vi "ZoneRed to ZoneBlue.vi"   [LabVIEW 2019]
uses:
  Global Var.vi
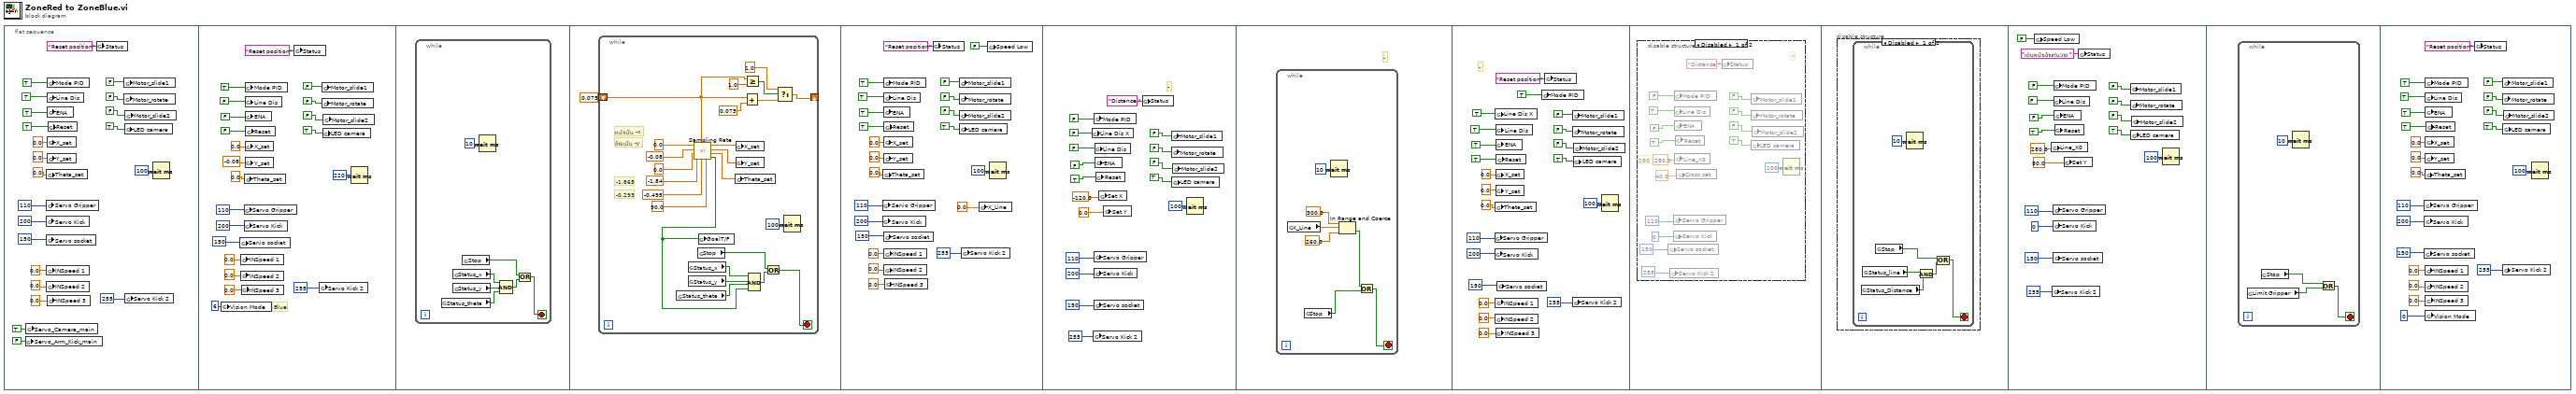
[diagram p0: block diagram]
diagram:
  n1 = flat-sequence {
    frame #0 {
      n2 = global write "Global Var.vi" "Servo_Arm_Kick_main"(FALSE ("Mode PID")) -> ()
      n3 = global write "Global Var.vi" "Servo_Camera_main"(TRUE ("Mode PID")) -> ()
      n4 = global write "Global Var.vi" "Servo Gripper"(u8 110 ("Servo Camera")) -> ()
      n5 = global write "Global Var.vi" "Servo Kick"(u8 200 ("Servo Camera")) -> ()
      n6 = global write "Global Var.vi" "Servo socket"(u8 150 ("Servo Camera")) -> ()
      n7 = global write "Global Var.vi" "Theta_set"(0.0 ("Theta_set")) -> ()
      n8 = global write "Global Var.vi" "INSpeed 1"(0.0 ("X_set")) -> ()
      n9 = global write "Global Var.vi" "INSpeed 2"(0.0 ("Y_set")) -> ()
      n10 = global write "Global Var.vi" "Mode PID"(TRUE ("Mode PID")) -> ()
      n11 = global write "Global Var.vi" "Line Dis"(TRUE ("Mode PID")) -> ()
      n12 = global write "Global Var.vi" "ENA"(TRUE ("ENA")) -> ()
      n13 = global write "Global Var.vi" "X_set"(0.0 ("X_set")) -> ()
      n14 = global write "Global Var.vi" "Y_set"(0.0 ("Y_set")) -> ()
      n15 = global write "Global Var.vi" "INSpeed 3"(0.0 ("Theta_set")) -> ()
      n16 = global write "Global Var.vi" "Reset"(TRUE ("ENA")) -> ()
      n17 = global write "Global Var.vi" "Status"("Reset position" ("Status")) -> ()
      n18 = global write "Global Var.vi" "Motor_slide1"(FALSE ("Mode PID")) -> ()
      n19 = global write "Global Var.vi" "Motor_rotate"(FALSE ("ENA")) -> ()
      n20 = global write "Global Var.vi" "LED camera"(TRUE ("LED camera")) -> ()
      n21 = global write "Global Var.vi" "Motor_slide2"(FALSE ("ENA")) -> ()
      n22 = global write "Global Var.vi" "Servo Kick 2"(u8 255 ("Servo Camera")) -> ()
      n23 = Wait (ms)(milliseconds to wait=u32 100) -> ()  [unwired: 1 out]
    }
    frame #1 {
      # "Blue"
      n24 = global write "Global Var.vi" "Vision Mode"(i16 6 ("Vision Mode")) -> ()
      n25 = global write "Global Var.vi" "Servo socket"(u8 150 ("Servo Camera")) -> ()
      n26 = global write "Global Var.vi" "INSpeed 1"(0.0 ("X_set")) -> ()
      n27 = global write "Global Var.vi" "INSpeed 2"(0.0 ("Y_set")) -> ()
      n28 = global write "Global Var.vi" "INSpeed 3"(0.0 ("Theta_set")) -> ()
      n29 = global write "Global Var.vi" "Servo Gripper"(u8 110 ("Servo Camera")) -> ()
      n30 = global write "Global Var.vi" "Servo Kick"(u8 200 ("Servo Camera")) -> ()
      n31 = global write "Global Var.vi" "Theta_set"(0.0 ("Theta_set")) -> ()
      n32 = global write "Global Var.vi" "Mode PID"(TRUE ("Mode PID")) -> ()
      n33 = global write "Global Var.vi" "Line Dis"(FALSE ("Mode PID")) -> ()
      n34 = global write "Global Var.vi" "ENA"(FALSE ("ENA")) -> ()
      n35 = global write "Global Var.vi" "X_set"(0.0 ("X_set")) -> ()
      n36 = global write "Global Var.vi" "Y_set"(-0.08 ("Y_set")) -> ()
      n37 = global write "Global Var.vi" "Reset"(FALSE ("ENA")) -> ()
      n38 = global write "Global Var.vi" "Status"("Reset position" ("Status")) -> ()
      n39 = global write "Global Var.vi" "Servo Kick 2"(u8 255 ("Servo Camera")) -> ()
      n40 = global write "Global Var.vi" "Motor_slide1"(FALSE ("Mode PID")) -> ()
      n41 = global write "Global Var.vi" "Motor_rotate"(FALSE ("ENA")) -> ()
      n42 = global write "Global Var.vi" "LED camera"(TRUE ("LED camera")) -> ()
      n43 = global write "Global Var.vi" "Motor_slide2"(FALSE ("ENA")) -> ()
      n44 = Wait (ms)(milliseconds to wait=u32 220) -> ()  [unwired: 1 out]
    }
    frame #2 {
      n45 = while {
        stop <- w46 stop-if-true
        n46 = global read "Global Var.vi" "Status_theta"() -> (w48:bool)
        n47 = global read "Global Var.vi" "Status_x"() -> (w49:bool)
        n48 = global read "Global Var.vi" "Status_y"() -> (w50:bool)
        n49 = global read "Global Var.vi" "Stop"() -> (w44:bool)
        n50 = Wait (ms)(milliseconds to wait=u32 10) -> ()  [unwired: 1 out]
        n51 = Compound Arithmetic op=AND(w49, w50, w48) -> (w45:bool)
        n52 = Or(x=w44, y=w45) -> (x .or. y?=w46:bool)
      }
    }
    frame #3 {
      n53 = while {
        shift-right: [w54] -> _
        shift-left: 0.075 -> [w52]
        stop <- w71 stop-if-true
        # "-0.293"
        # "-1.865"
        # "ซ้ายเป็น -y"
        # "หน้าเป็น -x"
        n54 = global read "Global Var.vi" "Status_theta"() -> (w73:bool)
        n55 = global read "Global Var.vi" "Status_x"() -> (w74:bool)
        n56 = global read "Global Var.vi" "Status_y"() -> (w75:bool)
        n57 = call "Sampling Rate.vi"("input a1"=90.0, "input y1"=-0.495, "T(0-1)"=w52, "input x1"=-1.84, "input a0"=0.0, "input y0"=-0.08, "input x0"=0.0) -> ("GoalT/F"=w59:bool, "a_output"=w66:dbl, "y_output"=w67:dbl, "x_output"=w68:dbl)  [unwired: 1 in]
        n58 = global read "Global Var.vi" "Stop"() -> (w69:bool)
        n59 = global write "Global Var.vi" "GoalT/F"(w59) -> ()
        n60 = global write "Global Var.vi" "Theta_set"(w66) -> ()
        n61 = global write "Global Var.vi" "X_set"(w68) -> ()
        n62 = global write "Global Var.vi" "Y_set"(w67) -> ()
        n63 = Add(x=w52, y=0.075) -> (x+y=w57:dbl)
        n64 = Greater Or Equal?(x=w52, y=1.0) -> (x >= y?=w56:bool)
        n65 = Compound Arithmetic op=AND(w74, w75, w73, w59) -> (w70:bool)
        n66 = Or(x=w69, y=w70) -> (x .or. y?=w71:bool)
        n67 = Select(t=1.0, s=w56, f=w57) -> (s? t:f=w54:dbl)
        n68 = Wait (ms)(milliseconds to wait=u32 100) -> ()  [unwired: 1 out]
      }
    }
    frame #4 {
      n69 = global write "Global Var.vi" "Servo Gripper"(u8 110 ("Servo Camera")) -> ()
      n70 = global write "Global Var.vi" "Servo Kick"(u8 200 ("Servo Camera")) -> ()
      n71 = global write "Global Var.vi" "Theta_set"(0.0 ("Theta_set")) -> ()
      n72 = global write "Global Var.vi" "Mode PID"(TRUE ("Mode PID")) -> ()
      n73 = global write "Global Var.vi" "Line Dis"(TRUE ("Mode PID")) -> ()
      n74 = global write "Global Var.vi" "ENA"(TRUE ("ENA")) -> ()
      n75 = global write "Global Var.vi" "X_set"(0.0 ("X_set")) -> ()
      n76 = global write "Global Var.vi" "Y_set"(0.0 ("Y_set")) -> ()
      n77 = global write "Global Var.vi" "Servo socket"(u8 150 ("Servo Camera")) -> ()
      n78 = global write "Global Var.vi" "Reset"(TRUE ("ENA")) -> ()
      n79 = global write "Global Var.vi" "INSpeed 1"(0.0 ("X_set")) -> ()
      n80 = global write "Global Var.vi" "INSpeed 2"(0.0 ("Y_set")) -> ()
      n81 = global write "Global Var.vi" "INSpeed 3"(0.0 ("Theta_set")) -> ()
      n82 = global write "Global Var.vi" "Status"("Reset position" ("Status")) -> ()
      n83 = global write "Global Var.vi" "Motor_slide1"(FALSE ("Mode PID")) -> ()
      n84 = global write "Global Var.vi" "Motor_rotate"(FALSE ("ENA")) -> ()
      n85 = global write "Global Var.vi" "Motor_slide2"(FALSE ("ENA")) -> ()
      n86 = global write "Global Var.vi" "LED camera"(TRUE ("LED camera")) -> ()
      n87 = global write "Global Var.vi" "Servo Kick 2"(u8 255 ("Servo Camera")) -> ()
      n88 = global write "Global Var.vi" "X_Line"(0.0 ("X_set")) -> ()
      n89 = global write "Global Var.vi" "Speed Low"(FALSE ("LED camera")) -> ()
      n90 = Wait (ms)(milliseconds to wait=u32 100) -> ()  [unwired: 1 out]
    }
    frame #5 {
      # "-"
      n91 = global write "Global Var.vi" "Line Dis X"(FALSE ("Mode PID")) -> ()
      n92 = global write "Global Var.vi" "Servo Kick 2"(u8 255 ("Servo Camera")) -> ()
      n93 = global write "Global Var.vi" "Mode PID"(FALSE ("Mode PID")) -> ()
      n94 = global write "Global Var.vi" "Servo Gripper"(u8 110 ("Servo Camera")) -> ()
      n95 = global write "Global Var.vi" "Servo Kick"(u8 200 ("Servo Camera")) -> ()
      n96 = global write "Global Var.vi" "Servo socket"(u8 150 ("Servo Camera")) -> ()
      n97 = global write "Global Var.vi" "Line Dis"(FALSE ("Mode PID")) -> ()
      n98 = global write "Global Var.vi" "ENA"(FALSE ("ENA")) -> ()
      n99 = global write "Global Var.vi" "Reset"(TRUE ("ENA")) -> ()
      n100 = global write "Global Var.vi" "Set X"(-120.0 ("Y_set")) -> ()
      n101 = global write "Global Var.vi" "Set Y"(0.0 ("Y_set")) -> ()
      n102 = global write "Global Var.vi" "Status"("Distance " ("Status")) -> ()
      n103 = global write "Global Var.vi" "Motor_slide1"(FALSE ("Mode PID")) -> ()
      n104 = global write "Global Var.vi" "Motor_rotate"(FALSE ("ENA")) -> ()
      n105 = global write "Global Var.vi" "LED camera"(TRUE ("LED camera")) -> ()
      n106 = global write "Global Var.vi" "Motor_slide2"(FALSE ("ENA")) -> ()
      n107 = Wait (ms)(milliseconds to wait=u32 100) -> ()  [unwired: 1 out]
    }
    frame #6 {
      # "-"
      n108 = while {
        stop <- w120 stop-if-true
        n109 = global read "Global Var.vi" "X_Line"() -> (w118:dbl)
        n110 = global read "Global Var.vi" "Stop"() -> (w119:bool)
        n111 = Wait (ms)(milliseconds to wait=u32 10) -> ()  [unwired: 1 out]
        n112 = In Range and Coerce(upper limit=300.0, x=w118, lower limit=260.0) -> (In Range?=w115:bool)  [unwired: 1 out]
        n113 = Or(x=w115, y=w119) -> (x .or. y?=w120:bool)
      }
    }
    frame #7 {
      # "-"
      n114 = global write "Global Var.vi" "Servo Gripper"(u8 110 ("Servo Camera")) -> ()
      n115 = global write "Global Var.vi" "Servo Kick"(u8 200 ("Servo Camera")) -> ()
      n116 = global write "Global Var.vi" "Line Dis X"(TRUE ("Mode PID")) -> ()
      n117 = global write "Global Var.vi" "Theta_set"(0.0 ("Theta_set")) -> ()
      n118 = global write "Global Var.vi" "INSpeed 1"(0.0 ("X_set")) -> ()
      n119 = global write "Global Var.vi" "INSpeed 2"(0.0 ("Y_set")) -> ()
      n120 = global write "Global Var.vi" "Line Dis"(TRUE ("Mode PID")) -> ()
      n121 = global write "Global Var.vi" "ENA"(TRUE ("ENA")) -> ()
      n122 = global write "Global Var.vi" "X_set"(0.0 ("X_set")) -> ()
      n123 = global write "Global Var.vi" "Y_set"(0.0 ("Y_set")) -> ()
      n124 = global write "Global Var.vi" "INSpeed 3"(0.0 ("Theta_set")) -> ()
      n125 = global write "Global Var.vi" "Reset"(TRUE ("ENA")) -> ()
      n126 = global write "Global Var.vi" "Servo socket"(u8 150 ("Servo Camera")) -> ()
      n127 = global write "Global Var.vi" "Mode PID"(TRUE ("Mode PID")) -> ()
      n128 = global write "Global Var.vi" "Status"("Reset position" ("Status")) -> ()
      n129 = global write "Global Var.vi" "Motor_slide1"(FALSE ("Mode PID")) -> ()
      n130 = global write "Global Var.vi" "Motor_rotate"(FALSE ("ENA")) -> ()
      n131 = global write "Global Var.vi" "Servo Kick 2"(u8 255 ("Servo Camera")) -> ()
      n132 = global write "Global Var.vi" "LED camera"(TRUE ("LED camera")) -> ()
      n133 = global write "Global Var.vi" "Motor_slide2"(FALSE ("ENA")) -> ()
      n134 = Wait (ms)(milliseconds to wait=u32 100) -> ()  [unwired: 1 out]
    }
    frame #8 {
      n135 = disable-structure shown="Disabled" {
        frame Disabled {
          # "280"
          # "*"
          n136 = global write "Global Var.vi" "Servo socket"(u8 150 ("Servo Camera")) -> ()
          n137 = global write "Global Var.vi" "Servo Kick 2"(u8 255 ("Servo Camera")) -> ()
          n138 = global write "Global Var.vi" "Servo Gripper"(u8 110 ("Servo Camera")) -> ()
          n139 = global write "Global Var.vi" "Servo Kick"(u8 0 ("Servo Camera")) -> ()
          n140 = global write "Global Var.vi" "Mode PID"(FALSE ("Mode PID")) -> ()
          n141 = global write "Global Var.vi" "Line Dis"(TRUE ("Mode PID")) -> ()
          n142 = global write "Global Var.vi" "ENA"(FALSE ("ENA")) -> ()
          n143 = global write "Global Var.vi" "Line_X0"(280.0 ("Y_set")) -> ()
          n144 = global write "Global Var.vi" "Reset"(TRUE ("ENA")) -> ()
          n145 = global write "Global Var.vi" "Cross set"(40.0 ("Y_set")) -> ()
          n146 = global write "Global Var.vi" "Status"("Distance " ("Status")) -> ()
          n147 = global write "Global Var.vi" "Motor_slide1"(FALSE ("Mode PID")) -> ()
          n148 = global write "Global Var.vi" "Motor_rotate"(FALSE ("ENA")) -> ()
          n149 = global write "Global Var.vi" "LED camera"(TRUE ("LED camera")) -> ()
          n150 = global write "Global Var.vi" "Motor_slide2"(FALSE ("ENA")) -> ()
          n151 = Wait (ms)(milliseconds to wait=u32 100) -> ()  [unwired: 1 out]
        }
        frame Enabled {
        }
      }
    }
    frame #9 {
      n152 = disable-structure shown="Disabled" {
        frame Disabled {
          n153 = while {
            stop <- w163 stop-if-true
            n154 = global read "Global Var.vi" "Status_Distance"() -> (w159:bool)
            n155 = global read "Global Var.vi" "Status_line"() -> (w160:bool)
            n156 = global read "Global Var.vi" "Stop"() -> (w162:bool)
            n157 = Wait (ms)(milliseconds to wait=u32 10) -> ()  [unwired: 1 out]
            n158 = And(x=w160, y=w159) -> (x .and. y?=w161:bool)
            n159 = Or(x=w162, y=w161) -> (x .or. y?=w163:bool)
          }
        }
        frame Enabled {
        }
      }
    }
    frame #10 {
      n160 = global write "Global Var.vi" "Speed Low"(FALSE ("LED camera")) -> ()
      n161 = global write "Global Var.vi" "Line_X0"(280.0 ("Y_set")) -> ()
      n162 = global write "Global Var.vi" "Servo Kick 2"(u8 255 ("Servo Camera")) -> ()
      n163 = global write "Global Var.vi" "Servo Gripper"(u8 110 ("Servo Camera")) -> ()
      n164 = global write "Global Var.vi" "Servo Kick"(u8 0 ("Servo Camera")) -> ()
      n165 = global write "Global Var.vi" "Servo socket"(u8 150 ("Servo Camera")) -> ()
      n166 = global write "Global Var.vi" "Mode PID"(FALSE ("Mode PID")) -> ()
      n167 = global write "Global Var.vi" "Line Dis"(FALSE ("Mode PID")) -> ()
      n168 = global write "Global Var.vi" "ENA"(FALSE ("ENA")) -> ()
      n169 = global write "Global Var.vi" "Reset"(TRUE ("ENA")) -> ()
      n170 = global write "Global Var.vi" "Set Y"(80.0 ("Y_set")) -> ()
      n171 = global write "Global Var.vi" "Status"("เดินหน้าเข้าแท่นวาง " ("Status")) -> ()
      n172 = global write "Global Var.vi" "Motor_slide1"(FALSE ("Mode PID")) -> ()
      n173 = global write "Global Var.vi" "Motor_rotate"(FALSE ("ENA")) -> ()
      n174 = global write "Global Var.vi" "LED camera"(TRUE ("LED camera")) -> ()
      n175 = global write "Global Var.vi" "Motor_slide2"(FALSE ("ENA")) -> ()
      n176 = Wait (ms)(milliseconds to wait=u32 100) -> ()  [unwired: 1 out]
    }
    frame #11 {
      n177 = while {
        stop <- w184 stop-if-true
        n178 = global read "Global Var.vi" "Limit Gripper"() -> (w182:bool)
        n179 = global read "Global Var.vi" "Stop"() -> (w183:bool)
        n180 = Wait (ms)(milliseconds to wait=u32 10) -> ()  [unwired: 1 out]
        n181 = Or(x=w183, y=w182) -> (x .or. y?=w184:bool)
      }
    }
    frame #12 {
      n182 = global write "Global Var.vi" "Servo Gripper"(u8 110 ("Servo Camera")) -> ()
      n183 = global write "Global Var.vi" "Servo Kick"(u8 200 ("Servo Camera")) -> ()
      n184 = global write "Global Var.vi" "Servo socket"(u8 150 ("Servo Camera")) -> ()
      n185 = global write "Global Var.vi" "Theta_set"(0.0 ("Theta_set")) -> ()
      n186 = global write "Global Var.vi" "INSpeed 1"(0.0 ("X_set")) -> ()
      n187 = global write "Global Var.vi" "INSpeed 2"(0.0 ("Y_set")) -> ()
      n188 = global write "Global Var.vi" "Mode PID"(TRUE ("Mode PID")) -> ()
      n189 = global write "Global Var.vi" "Line Dis"(TRUE ("Mode PID")) -> ()
      n190 = global write "Global Var.vi" "ENA"(TRUE ("ENA")) -> ()
      n191 = global write "Global Var.vi" "X_set"(0.0 ("X_set")) -> ()
      n192 = global write "Global Var.vi" "Y_set"(0.0 ("Y_set")) -> ()
      n193 = global write "Global Var.vi" "INSpeed 3"(0.0 ("Theta_set")) -> ()
      n194 = global write "Global Var.vi" "Vision Mode"(i16 0 ("Vision Mode")) -> ()
      n195 = global write "Global Var.vi" "Reset"(TRUE ("ENA")) -> ()
      n196 = global write "Global Var.vi" "Status"("Reset position" ("Status")) -> ()
      n197 = global write "Global Var.vi" "Motor_slide1"(FALSE ("Mode PID")) -> ()
      n198 = global write "Global Var.vi" "Motor_rotate"(FALSE ("ENA")) -> ()
      n199 = global write "Global Var.vi" "Servo Kick 2"(u8 255 ("Servo Camera")) -> ()
      n200 = global write "Global Var.vi" "LED camera"(TRUE ("LED camera")) -> ()
      n201 = global write "Global Var.vi" "Motor_slide2"(FALSE ("ENA")) -> ()
      n202 = Wait (ms)(milliseconds to wait=u32 100) -> ()  [unwired: 1 out]
    }
  }
